vi "Delete Element at Index.vi"(6 "index":i32, 8 "error in (no error)":errorcluster, 11 "Cluster in":variant) -> (0 "error out":errorcluster, 1 "element":variant, 2 "Name":string, 3 "Cluster out":variant)   [LabVIEW 2020, in "Variant Data Manipulation.lvlib"]
uses:
  Variant Data Manipulation.lvlib
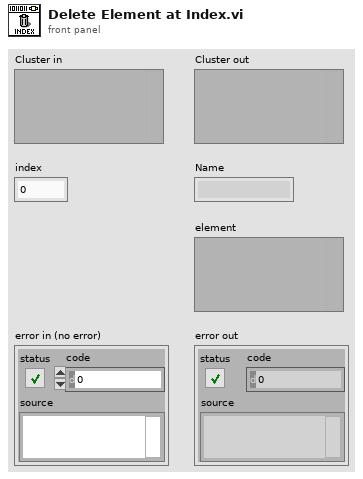
[diagram p1: front panel]
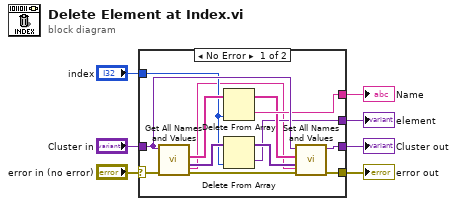
[diagram p0: block diagram]
diagram:
  n1 = case shown="No Error" "error in (no error)" {
    selector: "error in (no error)" -> [w20 w21]
    tunnel: [w17 w21] -> w6
    tunnel: [w16 w22] -> w5
    tunnel: "Cluster in" -> [w15 w22]
    tunnel: [w13 _] -> w3
    tunnel: [w10 _] -> w2
    tunnel: "index" -> [w9 _]
    frame No Error {
      n2 = call "Get All Names and Values.vi"("error in"=w20, "Cluster in"=w15) -> ("error out"=w18:errorcluster, "Values"=w19:variant[], "Element Names"=w14:string[], "Cluster Name"=w8:string)  [unwired: 5 in, 1 out]
      n3 = Delete From Array(array=w14, index=w9) -> (deleted portion=w13:string, array with subset deleted=w12:string[])  [unwired: 1 in]
      n4 = Delete From Array(array=w19, index=w9) -> (deleted portion=w10:variant, array with subset deleted=w11:variant[])  [unwired: 1 in]
      n5 = call "Set All Names and Values.vi"("Cluster Name"=w8, "error in"=w18, "values"=w11, "Element Names"=w12, "Cluster in"=w15) -> ("error out"=w17:errorcluster, "Cluster out"=w16:variant)  [unwired: 5 in]
    }
    frame Error {
    }
  }
  "Cluster out" <- w5
  "error out" <- w6
  "element" <- w2
  "Name" <- w3
